vi "CommonVIs_IsStringRepeatingItSelf.vi"(9 "Repeats(3)":u8=3, 10 "StateHistory":string[](array[string])) -> (2 "Repeating":bool)   [LabVIEW 2014]
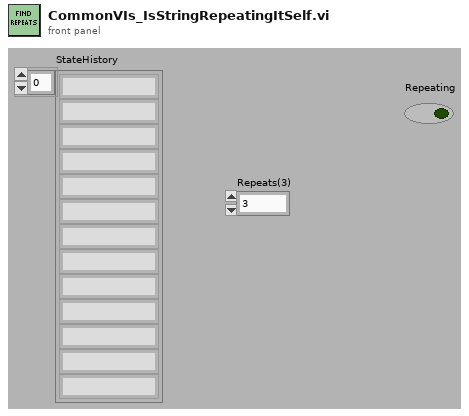
[diagram p1: front panel]
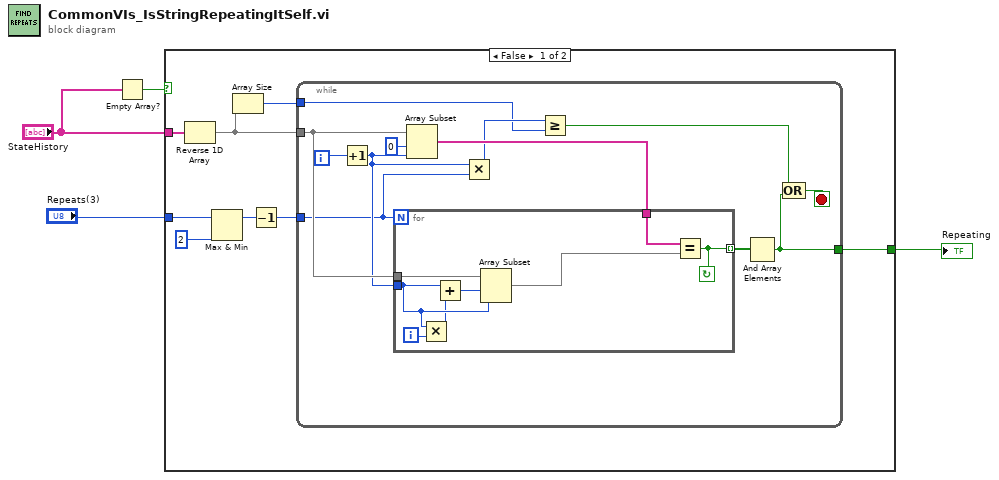
[diagram p0: block diagram]
diagram:
  n1 = Empty Array?(array="StateHistory") -> (empty?=w1:bool)
  n2 = case shown="False" w1 {
    tunnel: "Repeats(3)" -> [w12 _]
    tunnel: [w8 _] -> w3
    tunnel: "StateHistory" -> [w5 _]
    frame False {
      n3 = Reverse 1D Array(array=w5) -> (reversed array=w10:string[])
      n4 = Max & Min(x=w12, y=u8 2) -> (max(x,y)=w9:u8)  [unwired: 1 out]
      n5 = Array Size(array=w10) -> (size(s)=w6:i32)
      n6 = Decrement(x=w9) -> (x-1=w7:u8)
      n7 = while {
        tunnel: w10 -> [w22]
        tunnel: w7 -> [w16]
        tunnel: [w19] -> w8
        tunnel: w6 -> [w14]
        i -> [w24]
        stop <- w18 stop-if-true
        n8 = Increment(x=w24) -> (x+1=w17:i32)
        n9 = Array Subset(array=w22, index=0, length=w17) -> (w21:string[])
        n10 = for {
          N: w16 -> [_]
          tunnel: w22 -> [w31]
          tunnel: w21 -> [w32]
          tunnel: [w25] -> w20 mode=indexing
          tunnel: w17 -> [w28]
          i -> [w27]
          stop <- w25 continue-if-true
          n11 = Multiply(x=w28, y=w27) -> (x*y=w26:i32)
          n12 = Add(x=w28, y=w26) -> (x+y=w30:i32)
          n13 = Array Subset(array=w31, index=w30, length=w28) -> (w29:string[])
          n14 = Equal?(x=w32, y=w29) -> (x = y?=w25:bool)
        }
        n15 = Multiply(x=w17, y=w16) -> (x*y=w15:i32)
        n16 = Greater Or Equal?(x=w15, y=w14) -> (x >= y?=w13:bool)
        n17 = And Array Elements(Boolean array=w20) -> (logical AND=w19:bool)
        n18 = Compound Arithmetic op=OR(w13, w19) -> (w18:bool)
      }
    }
    frame True {
    }
  }
  "Repeating" <- w3
